vi "Update Facade.vi"(8 "Month Name":refnum<vi>, 9 "Dates":refnum<vi>, 10 "date time rec":T1, 11 "Display State In":cluster{"Month":i32, "Day":i32, "Year":i32}) -> ()   [LabVIEW 2019, in "Custom Calendar.xctl"]
uses:
  Custom Calendar.xctl
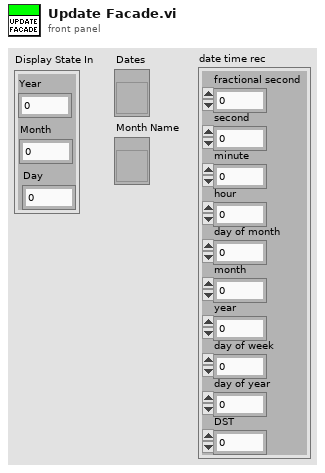
[diagram p1: front panel]
types:
  T1 = cluster{"fractional second":dbl, "second":i32, "minute":i32, "hour":i32, "day of month":i32, "month":i32, "year":i32, "day of week":i32, "day of year":i32, "DST":i32}
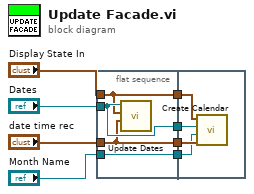
[diagram p0: block diagram]
diagram:
  n1 = flat-sequence {
    tunnel: "Display State In" -> [w10]
    tunnel: [w10] -> w7
    tunnel: "Dates" -> [w11]
    tunnel: "Month Name" -> [w12]
    tunnel: "date time rec" -> [w9]
    tunnel: [w11] -> w3
    tunnel: [w12] -> w2
    tunnel: [w9] -> w1
    tunnel: w7 -> [w16]
    tunnel: w3 -> [w13]
    tunnel: w2 -> [w14]
    tunnel: w1 -> [w15]
    frame #0 {
      n2 = call "Update Dates.vi"("date time rec"=w9, "Display State In"=w10, "Dates"=w11) -> ()  [unwired: 9 in]
    }
    frame #1 {
      n3 = call "Create Calendar.vi"("date time rec"=w15, "Month Name"=w14, "Dates"=w13, "Display State In"=w16) -> ()  [unwired: 8 in]
    }
  }
